vi "MockFAILC3.vi"(11 "MockFAILC3Settings":T1={"ModbusTxDataFIFO"="ModbusSubnetCTxDataFIFO", "Code17Memory"="MockFAILC3Code17", "BufferUpdateFIFO"="MockFAILC3Command", "ModbusRxDataFIFO"="ModbusSubnetCRxDataFIFO", "Code18Memory"="MockFAILC3Code18", "Code65Memory"="MockFAILC3Code65", "Code66Memory"="MockFAILC3Code66", "Code67Memory"="MockFAILC3Code67", "Code72Memory"="MockFAILC3Code72", "Code80Memory"="MockFAILC3Code80", "Code110Memory"="MockFAILC3Code110", "CRCDataFIFO"="MockFAILC3CRCDataFIFO", "CRCCalculateFIFO"="MockFAILC3CRCCalculateFIFO", "CRCFIFO"="MockFAILC3CRCFIFO"}) -> ()   [LabVIEW 2018, in "FPGAMockFAILC.lvlib"]
uses:
  FPGAMockFAILC.lvlib
  Common_FPGA_Modbus/DataTypes/ModbusCRCSettings.ctl
  DataTypes/MockFAILC3Settings.ctl
  Common_FPGA_Modbus/FPGAModbus.lvlib
panel:
  in  "ModbusCRCSettings":T2={"DataFIFO"="MockFAILC3CRCDataFIFO", "CalculateFIFO"="MockFAILC3CRCCalculateFIFO", "OutputFIFO"="MockFAILC3CRCFIFO"}
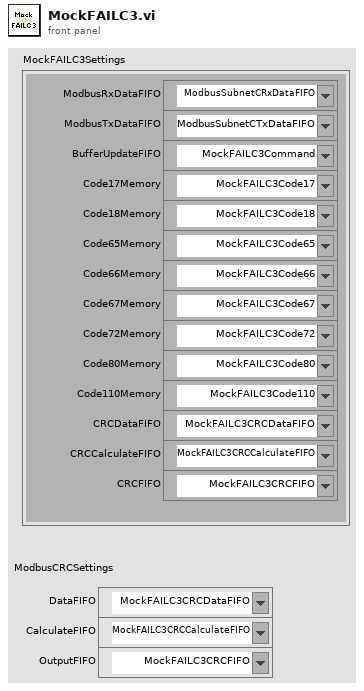
[diagram p1: front panel]
types:
  T1 = typedef "FPGAMockFAILC.lvlib/MockFAILC3Settings.ctl" = cluster{"ModbusTxDataFIFO":refnum<k21>, "Code17Memory":refnum<k21>, "BufferUpdateFIFO":refnum<k21>, "ModbusRxDataFIFO":refnum<k21>, "Code18Memory":refnum<k21>, "Code65Memory":refnum<k21>, "Code66Memory":refnum<k21>, "Code67Memory":refnum<k21>, "Code72Memory":refnum<k21>, "Code80Memory":refnum<k21>, "Code110Memory":refnum<k21>, "CRCDataFIFO":refnum<k21>, "CRCCalculateFIFO":refnum<k21>, "CRCFIFO":refnum<k21>}
  T2 = typedef "FPGAModbus.lvlib/ModbusCRCSettings.ctl" = cluster{"DataFIFO":refnum<k21>, "CalculateFIFO":refnum<k21>, "OutputFIFO":refnum<k21>}
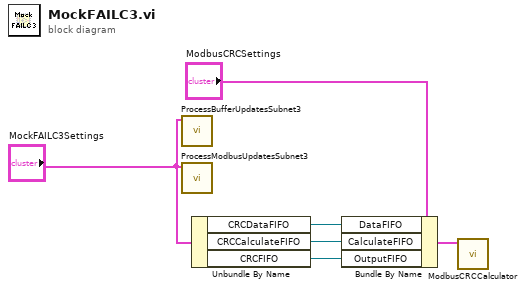
[diagram p0: block diagram]
diagram:
  n1 = call "ProcessBufferUpdatesSubnet3.vi"("MockFAILC3Settings"="MockFAILC3Settings") -> ()  [unwired: 11 in]
  n2 = call "ProcessModbusUpdatesSubnet3.vi"("MockFAILC3Settings"="MockFAILC3Settings") -> ()  [unwired: 11 in]
  n3 = Unbundle By Name("MockFAILC3Settings") -> ("CRCDataFIFO"=w3:refnum<k21>, "CRCCalculateFIFO"=w4:refnum<k21>, "CRCFIFO"=w5:refnum<k21>)
  n4 = Bundle By Name(cluster="ModbusCRCSettings", "DataFIFO"=w3, "CalculateFIFO"=w4, "OutputFIFO"=w5) -> (w6:T2)
  n5 = call "ModbusCRCCalculator.vi"("ModbusCRCSettings"=w6) -> ()  [unwired: 11 in]
